vi "TP 1.5.vi"() -> ()   [LabVIEW 2013]
panel:
  in  "F to C":bool caption="C  to F"
  out "Temperatura Convertida":dbl caption="[Cº]"
  in  "Temperatura Inicial":dbl caption="[Fº]"
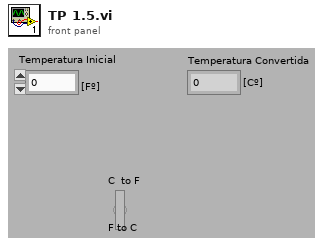
[diagram p1: front panel]
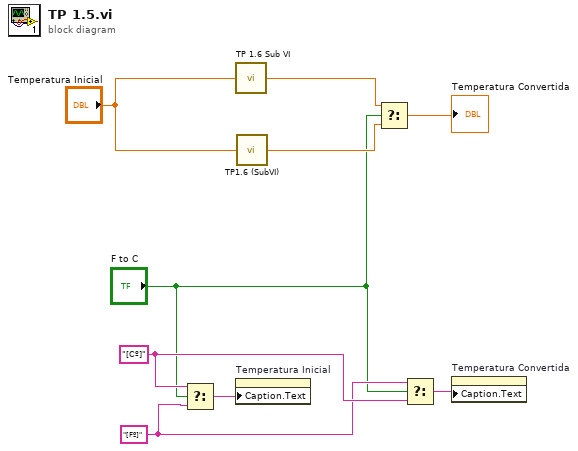
[diagram p0: block diagram]
diagram:
  w4 = "[Fº]"
  w5 = "[Cº]"
  n1 = Select(t=w5, s="F to C", f=w4) -> (s? t:f=w2:string)
  n2 = call "TP 1.6 Sub VI.vi"("Temp inicial"="Temperatura Inicial") -> ("Numeric"=w8:dbl)
  n3 = property on="Temperatura Inicial" class="DigNum (strict)"("Caption.Text"=w2) -> ()  [unwired: 2 in, 2 out]
  n4 = call "TP1.6 (SubVI).vi"("Temp inicial"="Temperatura Inicial") -> ("Numeric"=w7:dbl)
  n5 = Select(t=w8, s="F to C", f=w7) -> (s? t:f=→"Temperatura Convertida":dbl)
  n6 = Select(t=w4, s="F to C", f=w5) -> (s? t:f=w1:string)
  n7 = property on="Temperatura Convertida" class="DigNum (strict)"("Caption.Text"=w1) -> ()  [unwired: 2 in, 2 out]
